vi "DCDC_Model.vi"() -> ()   [LabVIEW 2017]
doc: "This example describes how to programmatically call a Model compiled by NI VeriStand and run this model in LabVIEW."
uses:
  <vilib>/Platform/TimedLoop/XDataNode/timing_clust.ctl
  <vilib>/Platform/TimedLoop/XDataNode/nitl_modes.ctl
  <vilib>/Platform/TimedLoop/XDataNode/wakeup.ctl
  <vilib>/Model Interface Toolkit/Model Interface Toolkit.lvclass/Model Interface Toolkit.ctl
  <vilib>/Model Interface Toolkit/Model Update.vi
  <vilib>/Model Interface Toolkit/Tick Model.vi
  <vilib>/Model Interface Toolkit/Probe Signals.vi
  <vilib>/Model Interface Toolkit/Multirate/Dispatch Model Tasks.vi
  <vilib>/Model Interface Toolkit/Call Model Start Routine.vi
  <vilib>/Model Interface Toolkit/Handle Error.vi
  <vilib>/Model Interface Toolkit/Multirate/Wait on Tasks.vi
  <vilib>/FPGAPlugInAG/myRIO-1900/niLvFpga_Open_myRIO-1900.vi
  <vilib>/rvi/interface/common/dynamic/niFpgaDynamicAddResources.vi
  <vilib>/Utility/error.llb/Error Cluster From Error Code.vi
  <vilib>/rvi/errors/niLvFpgaAdjustHostInterfaceError.vi
  <vilib>/Model Interface Toolkit/Check Error.vi
  <vilib>/Model Interface Toolkit/Generate Error Cluster.vi
  <vilib>/Platform/TimedLoop/scheduler/LVUserAPI/Fire Software-Triggered Timing Source.vi
  <vilib>/FPGAPlugInAG/Dynamic/niLvFpga_Close_Dynamic.vi
  <vilib>/Platform/TimedLoop/XDataNode/XDataNode.xnode
  <vilib>/rvi/interface/nirviOpenFPGA/nirviOpenFPGA.xnode
  FPGA Bitfiles/dcdcmyRIO2_FPGATarget_FPGAIO_Rf4SH5VSmXs.lvbitx
  FPGA_IO.vi
  <vilib>/rvi/interface/nirviReadWriteControl/nirviReadWriteControl.xnode
  <vilib>/rvi/interface/nirviCloseFPGA/nirviCloseFPGA.xnode
  <vilib>/Model Interface Toolkit/Model Interface Toolkit.lvclass
  <vilib>/Platform/TimedLoop/XDataNode/XDNodeRunTimeDep.lvlib
  <vilib>/rvi/interface/Simulation/niFpgaSimulationCallBeginRW.vi
  NiFpgaLv.dll
panel:
  out "U":dbl
  in  "Scale x2":dbl=10.0
  in  "Scale x1":dbl=5.0
  in  "Offset x2":dbl
  in  "Offset x1":dbl
  in  "x2_0":dbl=5.4
  in  "x1_0":dbl=0.7
  out "counter":dbl
  in  "SCOTS timestep":dbl=0.5
  out "x2":dbl
  out "x1":dbl
  in  "Chart History 3":i32=10000
  out "Input (from PFGA)":cluster{dbl[], dbl[]}(graph)
  out "Execution Time (ms)":u32
  out "Iteration":i32
  in  "clear":bool
  out "States":cluster{"x1":dbl[], "y1":dbl[]}[](graph)
  in  "Chart History 2":i32=10000
  in  "Chart History 1":i32=10000
  out "Voltage C":cluster{dbl[], dbl[]}(graph)
  out "Current L":cluster{dbl[], dbl[]}(graph)
  in  "Chart History 0":i32=10000
  out "Model Period (s)":dbl
  in  "stop":bool
  # "Overview: This test runs in only one MyRIO module. Simulink code is called every 5ms. Outputs and Inputs are sent/received every 0.5s\nRequirements: LabVIEW Model Interface Toolkit\nInstructions:\n1. Connect: AO0 <-> AI0, AO1 <-> AI1, DIO0 <-> DIO1 \n2. Run the FPGA controller code\n3. Run this VI"
  # "STATES CONVERSION"
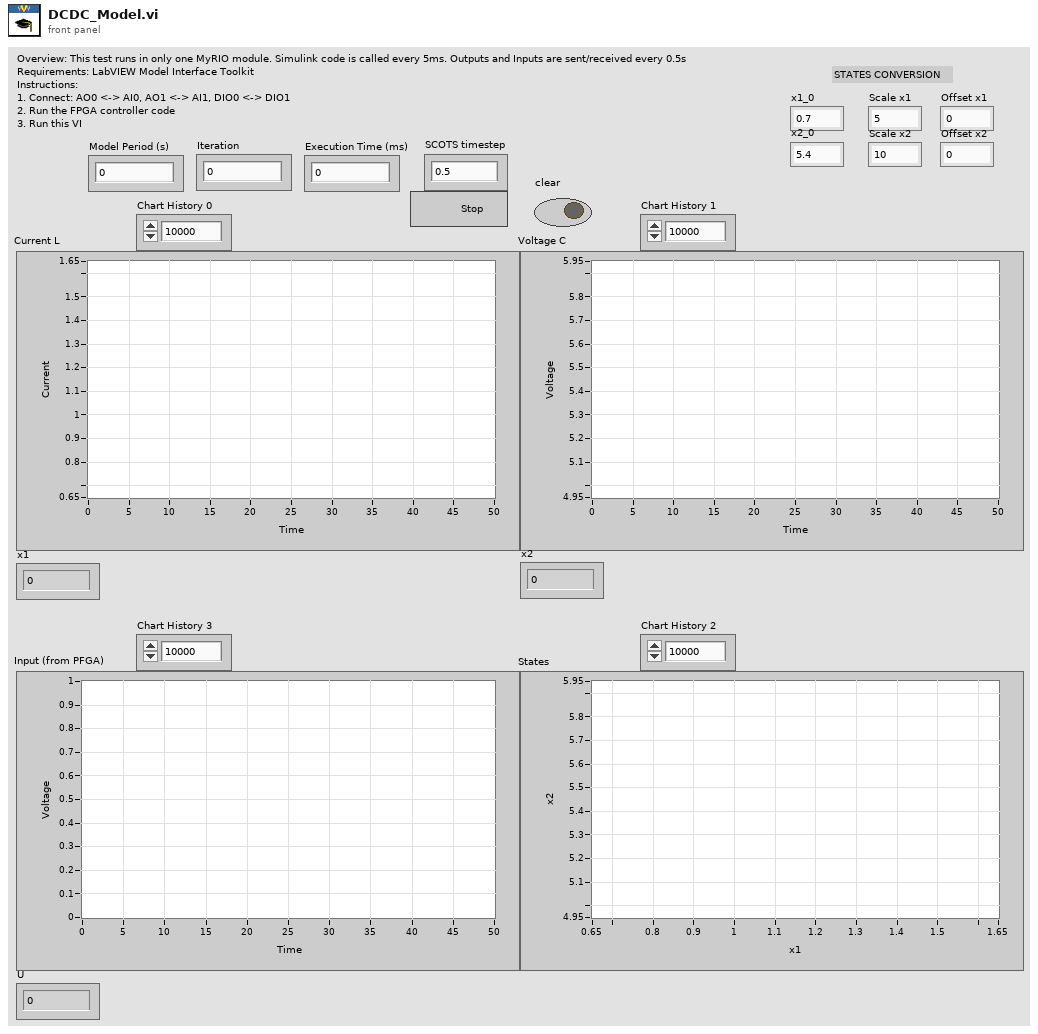
[diagram p1: front panel]
types:
  T1 = typedef "XDNodeRunTimeDep.lvlib/timing_clust.ctl" = cluster{"Expected End [f-1]":u64, "Actual End [f-1]":u64, "Finished Late? [f-1]":bool, "Expected End [i-1]":u64, "Actual End [i-1]":u64, "Finished Late? [i-1]":bool, "Expected Start [i]":u64, "Actual Start [i]":u64, "Expected Start [f]":u64, "Actual Start [f]":u64, "Source Name":string, "Structure Name":string, "Period":i64, "Deadline":i64, "Offset":i64, "Start":i64, "Priority":i32, "Timeout":i32, "Mode":T2, "Wakeup Reason":T3, "Error":errorcluster, "Source Type":string, "Secondary Source Type":string, "Global End Time":u64, "Global Start Time":u64, "Frame Duration":u64, "Iteration Duration":u64, "Assigned CPU":i32, "I/O Scan Engine Mode":u32}
  T2 = typedef "XDNodeRunTimeDep.lvlib/nitl_modes.ctl" = enum32{"No Change", "Process missed periods, maintain original phase", "Discard missed periods, maintain original phase", "Process missed periods, ignore original phase", "Discard missed periods, ignore original phase"}
  T3 = typedef "XDNodeRunTimeDep.lvlib/wakeup.ctl" = enum32{"Normal", "Aborted", "Asynchronous wakeup", "Timing source error", "Timed loop error", "Timeout"}
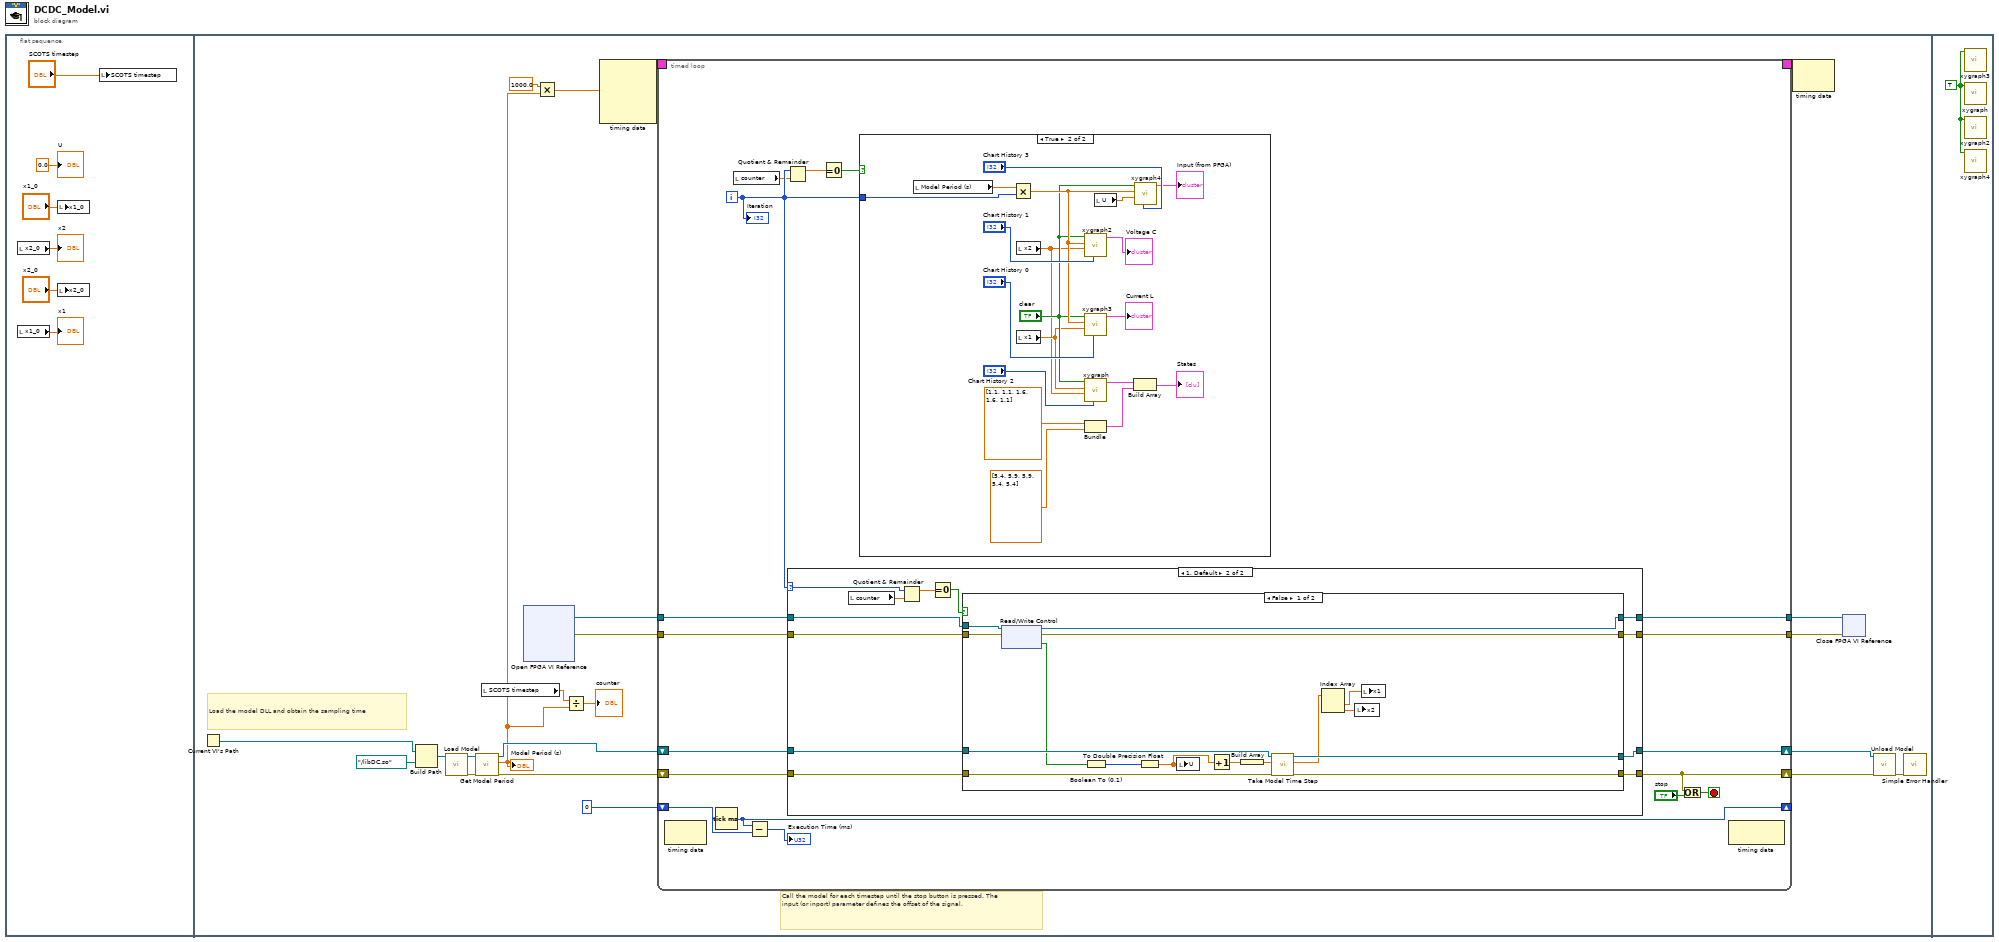
[diagram p0: block diagram]
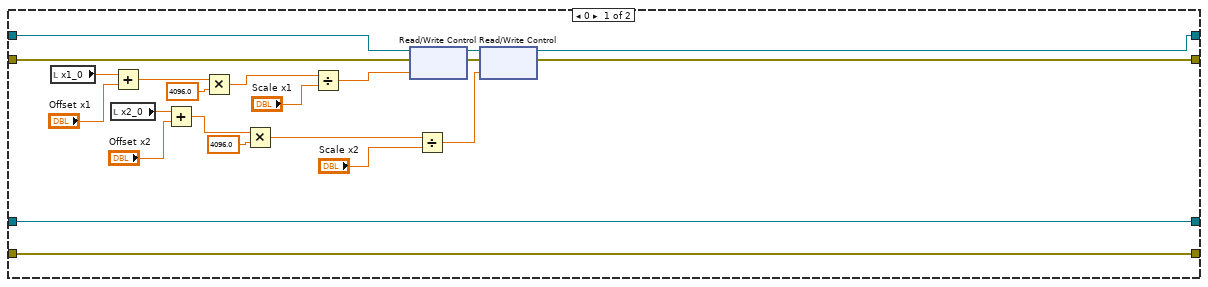
[diagram p3: hidden frame]
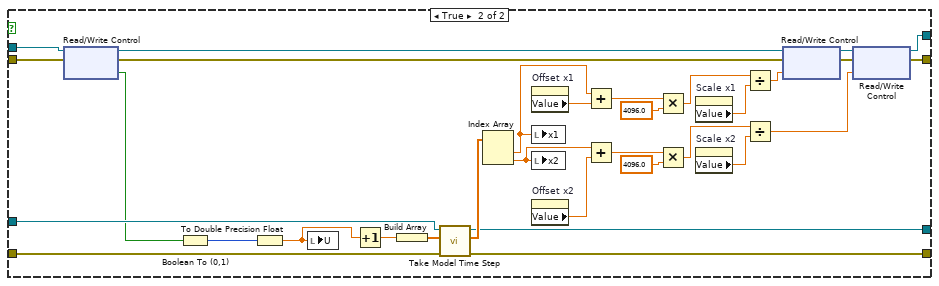
[diagram p4: hidden frame]
diagram:
  n1 = flat-sequence {
    frame #0 {
      n2 = local read "x2_0"() -> (→"x2":dbl)
      n3 = local read "x1_0"() -> (→"x1":dbl)
      n4 = local write "x1_0"("x1_0") -> ()
      n5 = local write "x2_0"("x2_0") -> ()
      n6 = local write "SCOTS timestep"("SCOTS timestep") -> ()
      "U" <- 0.0
    }
    frame #1 {
      # "Call the model for each timestep until the stop button is pressed. The input (or inport) parameter defines the offset of the signal."
      # "Load the model DLL and obtain the sampling time"
      n7 = Current VI's Path() -> (path=w25:path)
      n8 = Build Path(base path=w25, name or relative path=path "../libDC.so" ("Model Path")) -> (appended path=w26:path)
      n9 = call <vilib>:"Load Model.vi"("Model Path"=w26) -> ("error out"=w23:errorcluster, "Model out"=w17:refnum<class "Model Interface Toolkit.lvclass">)  [unwired: 9 in]
      n10 = call <vilib>:"Get Model Period.vi"("error in"=w23, "Model in"=w17) -> ("error out"=w19:errorcluster, "Model Period (s)"=w7:dbl, "Model out"=w21:refnum<class "Model Interface Toolkit.lvclass">)  [unwired: 7 in]
      "Model Period (s)" <- w7
      n11 = local read "SCOTS timestep"() -> (w8:dbl)
      n12 = xnode "Open FPGA VI Reference"() -> ("FPGA VI Reference Out"=w14:refnum<k20>, "error out"=w13:errorcluster)  [unwired: 2 in]
      n13 = Multiply(x=1000.0, y=w7) -> (x*y=w22:dbl)
      n14 = Divide(x=w8, y=w7) -> (x/y=→"counter":dbl)
      n15 = node-c288(w22) -> (w28:T1)  [unwired: 3 in]
      n16 = timed-loop {
        timing: w28 -> [_]
        timing-out: [_] -> w27
        shift-right: [w44] -> w20
        shift-left: w21 -> [w45]
        shift-right: [w40] -> w18
        shift-left: w19 -> [w43]
        tunnel: w14 -> [w37]
        tunnel: w13 -> [w36]
        tunnel: [w35] -> w12
        tunnel: [w34] -> w11
        shift-right: [w33] -> _
        shift-left: 0 -> [w32]
        i -> [w31]
        stop <- w41 stop-if-true
        n17 = node-c288() -> ()  [unwired: 1 in, 1 out]
        n18 = Tick Count (ms)() -> (millisecond timer value=w33:u32)
        n19 = local read "counter"() -> (w29:dbl)
        n20 = Subtract(x=w33, y=w32) -> (x-y=→"Execution Time (ms)":u32)
        n21 = Quotient & Remainder(x=w31, y=w29) -> (x-y*floor(x/y)=w39:dbl)  [unwired: 1 out]
        n22 = case shown="1, Default" w31 {
          selector: w31 -> [_ w92]
          tunnel: w45 -> [w86 w98]
          tunnel: [w86 w96] -> w44
          tunnel: w43 -> [w85 w95]
          tunnel: [w85 w97] -> w40
          tunnel: w37 -> [w81 w91]
          tunnel: w36 -> [w80 w90]
          tunnel: [w74 w89] -> w35
          tunnel: [w73 w88] -> w34
          frame 0 {
            n23 = local read "x1_0"() -> (w70:dbl)
            n24 = local read "x2_0"() -> (w67:dbl)
            n25 = Add(x=w70, y="Offset x1") -> (x+y=w69:dbl)
            n26 = Add(x=w67, y="Offset x2") -> (x+y=w65:dbl)
            n27 = Multiply(x=w69, y=sgl 4096.0 ("Slide")) -> (x*y=w84:dbl)
            n28 = Multiply(x=w65, y=sgl 4096.0 ("Slide")) -> (x*y=w77:dbl)
            n29 = Divide(x=w84, y="Scale x1") -> (x/y=w82:dbl)
            n30 = xnode "Read/Write Control"("FPGA VI Reference In"=w81, "error in"=w80, "x1_read"=w82) -> ("FPGA VI Reference Out"=w79:refnum<k20>, "error out"=w78:errorcluster)
            n31 = Divide(x=w77, y="Scale x2") -> (x/y=w75:dbl)
            n32 = xnode "Read/Write Control"("FPGA VI Reference In"=w79, "error in"=w78, "x2_read"=w75) -> ("FPGA VI Reference Out"=w74:refnum<k20>, "error out"=w73:errorcluster)
          }
          frame 1, Default {
            n33 = local read "counter"() -> (w87:dbl)
            n34 = Quotient & Remainder(x=w92, y=w87) -> (x-y*floor(x/y)=w93:dbl)  [unwired: 1 out]
            n35 = Equal To 0?(x=w93) -> (x = 0?=w94:bool)
            n36 = case shown="False" w94 {
              tunnel: w98 -> [w114 w142]
              tunnel: [w112 w141] -> w97
              tunnel: [w113 w140] -> w96
              tunnel: w95 -> [w111 w139]
              tunnel: w91 -> [w104 w138]
              tunnel: w90 -> [w107 w131]
              tunnel: [w105 w135] -> w89
              tunnel: [w106 w134] -> w88
              frame False {
                n37 = xnode "Read/Write Control"("FPGA VI Reference In"=w104, "error in"=w107) -> ("FPGA VI Reference Out"=w105:refnum<k20>, "error out"=w106:errorcluster, "U_read"=w103:bool)
                n38 = Boolean To (0,1)(Boolean=w103) -> (0, 1=w109:i16)
                n39 = To Double Precision Float(number=w109) -> (double precision float=w102:dbl)
                n40 = local write "U"(w102) -> ()
                n41 = Increment(x=w102) -> (x+1=w110:dbl)
                n42 = Build Array(w110) -> (w108:dbl[])
                n43 = call <vilib>:"Take Model Time Step.vi"("error in (no error)"=w111, "Inport Array"=w108, "Model in"=w114) -> ("error out"=w112:errorcluster, "Outport Array out"=w101:dbl[], "Model out"=w113:refnum<class "Model Interface Toolkit.lvclass">)  [unwired: 6 in]
                n44 = Index Array(array=w101) -> (element #1=w100:dbl, element #2=w99:dbl)  [unwired: 2 in]
                n45 = local write "x2"(w99) -> ()
                n46 = local write "x1"(w100) -> ()
              }
              frame True {
                n47 = xnode "Read/Write Control"("FPGA VI Reference In"=w138, "error in"=w131) -> ("FPGA VI Reference Out"=w137:refnum<k20>, "error out"=w132:errorcluster, "U_read"=w130:bool)
                n48 = Boolean To (0,1)(Boolean=w130) -> (0, 1=w145:i16)
                n49 = To Double Precision Float(number=w145) -> (double precision float=w115:dbl)
                n50 = local write "U"(w115) -> ()
                n51 = Increment(x=w115) -> (x+1=w146:dbl)
                n52 = Build Array(w146) -> (w144:dbl[])
                n53 = call <vilib>:"Take Model Time Step.vi"("error in (no error)"=w139, "Inport Array"=w144, "Model in"=w142) -> ("error out"=w141:errorcluster, "Outport Array out"=w143:dbl[], "Model out"=w140:refnum<class "Model Interface Toolkit.lvclass">)  [unwired: 6 in]
                n54 = Index Array(array=w143) -> (element #1=w123:dbl, element #2=w118:dbl)  [unwired: 2 in]
                n55 = property on="Offset x1" class="DigNum (strict)"() -> ("Value"=w122:dbl)  [unwired: 2 in, 2 out]
                n56 = local write "x1"(w123) -> ()
                n57 = local write "x2"(w118) -> ()
                n58 = property on="Offset x2" class="DigNum (strict)"() -> ("Value"=w117:dbl)  [unwired: 2 in, 2 out]
                n59 = Add(x=w123, y=w122) -> (x+y=w125:dbl)
                n60 = Add(x=w118, y=w117) -> (x+y=w124:dbl)
                n61 = Multiply(x=w125, y=sgl 4096.0 ("Slide")) -> (x*y=w129:dbl)
                n62 = Multiply(x=w124, y=sgl 4096.0 ("Slide")) -> (x*y=w127:dbl)
                n63 = property on="Scale x1" class="DigNum (strict)"() -> ("Value"=w121:dbl)  [unwired: 2 in, 2 out]
                n64 = property on="Scale x2" class="DigNum (strict)"() -> ("Value"=w119:dbl)  [unwired: 2 in, 2 out]
                n65 = Divide(x=w129, y=w121) -> (x/y=w120:dbl)
                n66 = Divide(x=w127, y=w119) -> (x/y=w116:dbl)
                n67 = xnode "Read/Write Control"("FPGA VI Reference In"=w137, "error in"=w132, "x1_read"=w120) -> ("FPGA VI Reference Out"=w136:refnum<k20>, "error out"=w133:errorcluster)
                n68 = xnode "Read/Write Control"("FPGA VI Reference In"=w136, "error in"=w133, "x2_read"=w116) -> ("FPGA VI Reference Out"=w135:refnum<k20>, "error out"=w134:errorcluster)
              }
            }
          }
        }
        n69 = Equal To 0?(x=w39) -> (x = 0?=w38:bool)
        n70 = case shown="True" w38 {
          tunnel: w31 -> [_ w52]
          frame False {
          }
          frame True {
            n71 = local read "Model Period (s)"() -> (w49:dbl)
            n72 = Multiply(x=w49, y=w52) -> (x*y=w51:dbl)
            n73 = local read "x2"() -> (w46:dbl)
            n74 = local read "x1"() -> (w47:dbl)
            n75 = call "xygraph2.vi"("Chart History (10,000)"="Chart History 1", "Y Value"=w46, "X Value"=w51, "clear 2"="clear") -> ("Cluster"=→"Voltage C":cluster{dbl[], dbl[]})  [unwired: 7 in]
            n76 = call "xygraph3.vi"("Chart History (10,000)"="Chart History 0", "Y Value"=w47, "X Value"=w51, "clear"="clear") -> ("Cluster"=→"Current L":cluster{dbl[], dbl[]})  [unwired: 7 in]
            n77 = call "xygraph.vi"("Chart History (10,000)"="Chart History 2", "Y Value"=w46, "X Value"=w47, "clear 1"="clear") -> ("Cluster"=w57:cluster{dbl[], dbl[]})  [unwired: 7 in]
            n78 = Bundle("x1"=dbl[] [1.1, 1.1, 1.6, 1.6, 1.1], "y1"=dbl[] [5.4, 5.9, 5.9, 5.4, 5.4]) -> (w55:cluster{"x1":dbl[], "y1":dbl[]})  [unwired: 1 in]
            n79 = local read "U"() -> (w48:dbl)
            n80 = Build Array(w57, w55) -> (→"States":cluster{"x1":dbl[], "y1":dbl[]}[])
            n81 = call "xygraph4.vi"("Chart History (10,000)"="Chart History 3", "Y Value"=w48, "X Value"=w51, "clear"="clear") -> ("Cluster"=→"Input (from PFGA)":cluster{dbl[], dbl[]})  [unwired: 7 in]
          }
        }
        n82 = Or(x=w40, y="stop") -> (x .or. y?=w41:bool)
        n83 = node-c288() -> ()  [unwired: 1 in, 1 out]
        "Iteration" <- w31
      }
      n84 = node-c288(w27) -> ()  [unwired: 1 out]
      n85 = xnode "Close FPGA VI Reference"("FPGA VI Reference In"=w12, "error in"=w11) -> ()  [unwired: 1 out]
      n86 = call <vilib>:"Unload Model.vi"("error in (no error)"=w18, "Model in"=w20) -> ("error out"=w16:errorcluster)  [unwired: 9 in]
      n87 = call <vilib>:"Simple Error Handler.vi"("error in (no error)"=w16) -> ()  [unwired: 4 in, 5 out]
    }
    frame #2 {
      w153 = TRUE
      n88 = call "xygraph3.vi"("clear"=w153) -> ()  [unwired: 10 in, 1 out]
      n89 = call "xygraph.vi"("clear 1"=w153) -> ()  [unwired: 10 in, 1 out]
      n90 = call "xygraph2.vi"("clear 2"=w153) -> ()  [unwired: 10 in, 1 out]
      n91 = call "xygraph4.vi"("clear"=w153) -> ()  [unwired: 10 in, 1 out]
    }
  }
